vi "AKD Get Motor IPeak.vi"(0 "connection ID":refnum<k5>, 11 "error in":errorcluster) -> (4 "TCP Refnum":refnum<k5>, 6 "motor IPeak (Arms)":sgl, 15 "error out":errorcluster)   [LabVIEW 2019]
doc: "This VI gets the value of motor peak current (Arms) stored in the AKD drive."
uses:
  MODBUS/NI Modbus.llb/MB Ethernet Master Query Read Holding Registers (poly).vi
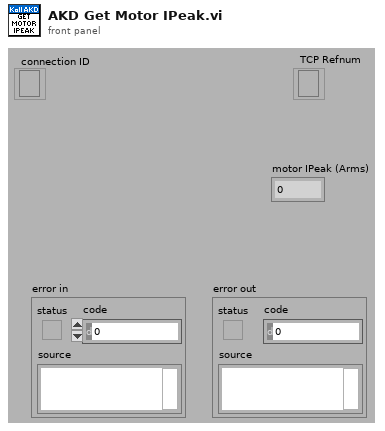
[diagram p1: front panel]
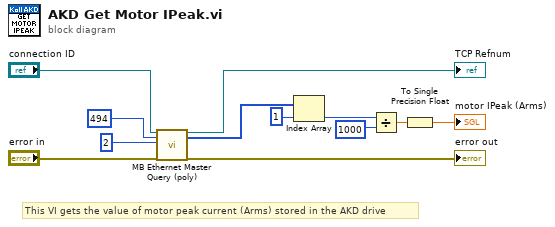
[diagram p0: block diagram]
diagram:
  # "This VI gets the value of motor peak current (Arms) stored in the AKD drive"
  n1 = call-poly "MB Ethernet Master Query (poly).vi"("TCP Connection Refnum in"="connection ID", "Starting Address"=u16 494, "Quantity"=u16 2, "error in"="error in") -> ("TCP Connection Refnum (dup)"=→"TCP Refnum":refnum<k5>, "Holding Registers"=w2:u16[], "error out"=→"error out":errorcluster)  [unwired: 12 in, 1 out]
  n2 = Index Array(array=w2, index=1) -> (element=w5:u16)
  n3 = Divide(x=w5, y=u16 1000) -> (x/y=w3:dbl)
  n4 = To Single Precision Float(number=w3) -> (single precision float=→"motor IPeak (Arms)":sgl)
